vi "Lab Panel V6.00.vi"() -> ()   [LabVIEW 2017] (continued)
                            n1487 = local write "DISP LAB03-1"(w2783) -> ()
                          }
                        }
                      }
                      frame False {
                      }
                    }
                  }
                }
              }
              frame #5 {
                # "LAB03-2"
                n1488 = Equal?(x=w2786, y=2) -> (x = y?=w2789:bool)
                n1489 = local read "DISP LAB03-2"() -> (w2791:T4)
                n1490 = Unbundle(w2791) -> ("STATUS"=w2792:string)  [unwired: 2 out]
                n1491 = Equal?(x=w2792, y="RUN") -> (x = y?=w2788:bool)
                n1492 = And(x=w2788, y=w2789) -> (x .and. y?=w2787:bool)
                n1493 = case shown="True" w2787 {
                  tunnel: w2791 -> [_ w2795]
                  tunnel: w2785 -> [_ w2798]
                  frame False {
                  }
                  frame True {
                    n1494 = local read "SET LAB03-2"() -> (w2797:T5)
                    n1495 = local read "TDMS LAB03-2"() -> (w2794:refnum<k34>)
                    n1496 = Unbundle(w2795) -> ("CYCLE"=w2799:dbl)  [unwired: 2 out]
                    n1497 = Unbundle(w2797) -> ("T-RISE mins"=w2796:dbl)  [unwired: 4 out]
                    n1498 = Greater Or Equal?(x=w2799, y=w2798) -> (x >= y?=w2800:bool)
                    n1499 = case shown="True" w2800 {
                      tunnel: w2796 -> [w2803 _]
                      tunnel: w2795 -> [w2802 _]
                      tunnel: w2794 -> [w2801 _]
                      frame True {
                        n1500 = stacked-sequence {
                          tunnel: w2803 -> [w2806 _]
                          tunnel: w2802 -> [_ w2811]
                          tunnel: w2801 -> [w2804 _]
                          frame #0 {
                            n1501 = Build Array("T-RISE") -> (w2808:string[])
                            n1502 = Build Array(w2806) -> (w2807:dbl[])
                            n1503 = TDMS Write(0:w2804, 5:"TEST PASS", 7:w2808, 9:w2807) -> (15:w2810:errorcluster)  [unwired: 2 in, 3 out]
                            n1504 = local write "data file error"(w2810) -> ()
                          }
                          frame #1 {
                            n1505 = Bundle(cluster=w2811, "STATUS"="T-RISE PASS") -> (w2813:T4)  [unwired: 2 in]
                            n1506 = local write "RESULT LAB03-2"(TRUE) -> ()
                            n1507 = local write "DISP LAB03-2"(w2813) -> ()
                          }
                        }
                      }
                      frame False {
                      }
                    }
                  }
                }
              }
              frame #6 {
                # "LAB04-1"
                n1508 = Equal?(x=w2816, y=2) -> (x = y?=w2819:bool)
                n1509 = local read "DISP LAB04-1"() -> (w2821:T4)
                n1510 = Unbundle(w2821) -> ("STATUS"=w2822:string)  [unwired: 2 out]
                n1511 = Equal?(x=w2822, y="RUN") -> (x = y?=w2818:bool)
                n1512 = And(x=w2818, y=w2819) -> (x .and. y?=w2817:bool)
                n1513 = case shown="True" w2817 {
                  tunnel: w2821 -> [_ w2825]
                  tunnel: w2815 -> [_ w2828]
                  frame False {
                  }
                  frame True {
                    n1514 = local read "SET LAB04-1"() -> (w2827:T5)
                    n1515 = local read "TDMS LAB04-1"() -> (w2824:refnum<k34>)
                    n1516 = Unbundle(w2825) -> ("CYCLE"=w2829:dbl)  [unwired: 2 out]
                    n1517 = Unbundle(w2827) -> ("T-RISE mins"=w2826:dbl)  [unwired: 4 out]
                    n1518 = Greater Or Equal?(x=w2829, y=w2828) -> (x >= y?=w2830:bool)
                    n1519 = case shown="True" w2830 {
                      tunnel: w2826 -> [w2833 _]
                      tunnel: w2825 -> [w2832 _]
                      tunnel: w2824 -> [w2831 _]
                      frame True {
                        n1520 = stacked-sequence {
                          tunnel: w2833 -> [w2836 _]
                          tunnel: w2832 -> [_ w2841]
                          tunnel: w2831 -> [w2834 _]
                          frame #0 {
                            n1521 = Build Array("T-RISE") -> (w2838:string[])
                            n1522 = Build Array(w2836) -> (w2837:dbl[])
                            n1523 = TDMS Write(0:w2834, 5:"TEST PASS", 7:w2838, 9:w2837) -> (15:w2840:errorcluster)  [unwired: 2 in, 3 out]
                            n1524 = local write "data file error"(w2840) -> ()
                          }
                          frame #1 {
                            n1525 = Bundle(cluster=w2841, "STATUS"="T-RISE PASS") -> (w2843:T4)  [unwired: 2 in]
                            n1526 = local write "RESULT LAB04-1"(TRUE) -> ()
                            n1527 = local write "DISP LAB04-1"(w2843) -> ()
                          }
                        }
                      }
                      frame False {
                      }
                    }
                  }
                }
              }
              frame #7 {
                # "LAB04-2"
                n1528 = Equal?(x=w2846, y=2) -> (x = y?=w2849:bool)
                n1529 = local read "DISP LAB04-2"() -> (w2851:T4)
                n1530 = Unbundle(w2851) -> ("STATUS"=w2852:string)  [unwired: 2 out]
                n1531 = Equal?(x=w2852, y="RUN") -> (x = y?=w2848:bool)
                n1532 = And(x=w2848, y=w2849) -> (x .and. y?=w2847:bool)
                n1533 = case shown="True" w2847 {
                  tunnel: w2851 -> [_ w2855]
                  tunnel: w2845 -> [_ w2858]
                  frame False {
                  }
                  frame True {
                    n1534 = local read "SET LAB04-2"() -> (w2857:T5)
                    n1535 = local read "TDMS LAB04-2"() -> (w2854:refnum<k34>)
                    n1536 = Unbundle(w2855) -> ("CYCLE"=w2859:dbl)  [unwired: 2 out]
                    n1537 = Unbundle(w2857) -> ("T-RISE mins"=w2856:dbl)  [unwired: 4 out]
                    n1538 = Greater Or Equal?(x=w2859, y=w2858) -> (x >= y?=w2860:bool)
                    n1539 = case shown="True" w2860 {
                      tunnel: w2856 -> [w2863 _]
                      tunnel: w2855 -> [w2862 _]
                      tunnel: w2854 -> [w2861 _]
                      frame True {
                        n1540 = stacked-sequence {
                          tunnel: w2863 -> [w2866 _]
                          tunnel: w2862 -> [_ w2871]
                          tunnel: w2861 -> [w2864 _]
                          frame #0 {
                            n1541 = Build Array("T-RISE") -> (w2868:string[])
                            n1542 = Build Array(w2866) -> (w2867:dbl[])
                            n1543 = TDMS Write(0:w2864, 5:"TEST PASS", 7:w2868, 9:w2867) -> (15:w2870:errorcluster)  [unwired: 2 in, 3 out]
                            n1544 = local write "data file error"(w2870) -> ()
                          }
                          frame #1 {
                            n1545 = Bundle(cluster=w2871, "STATUS"="T-RISE PASS") -> (w2873:T4)  [unwired: 2 in]
                            n1546 = local write "RESULT LAB04-2"(TRUE) -> ()
                            n1547 = local write "DISP LAB04-2"(w2873) -> ()
                          }
                        }
                      }
                      frame False {
                      }
                    }
                  }
                }
              }
              frame #8 {
                # "LAB05-1"
                n1548 = Equal?(x=w2876, y=2) -> (x = y?=w2879:bool)
                n1549 = local read "DISP LAB05-1"() -> (w2881:T4)
                n1550 = Unbundle(w2881) -> ("STATUS"=w2882:string)  [unwired: 2 out]
                n1551 = Equal?(x=w2882, y="RUN") -> (x = y?=w2878:bool)
                n1552 = And(x=w2878, y=w2879) -> (x .and. y?=w2877:bool)
                n1553 = case shown="True" w2877 {
                  tunnel: w2881 -> [_ w2885]
                  tunnel: w2875 -> [_ w2888]
                  frame False {
                  }
                  frame True {
                    n1554 = local read "SET LAB05-1"() -> (w2887:T5)
                    n1555 = local read "TDMS LAB05-1"() -> (w2884:refnum<k34>)
                    n1556 = Unbundle(w2885) -> ("CYCLE"=w2889:dbl)  [unwired: 2 out]
                    n1557 = Unbundle(w2887) -> ("T-RISE mins"=w2886:dbl)  [unwired: 4 out]
                    n1558 = Greater Or Equal?(x=w2889, y=w2888) -> (x >= y?=w2890:bool)
                    n1559 = case shown="True" w2890 {
                      tunnel: w2886 -> [w2893 _]
                      tunnel: w2885 -> [w2892 _]
                      tunnel: w2884 -> [w2891 _]
                      frame True {
                        n1560 = stacked-sequence {
                          tunnel: w2893 -> [w2896 _]
                          tunnel: w2892 -> [_ w2901]
                          tunnel: w2891 -> [w2894 _]
                          frame #0 {
                            n1561 = Build Array("T-RISE") -> (w2898:string[])
                            n1562 = Build Array(w2896) -> (w2897:dbl[])
                            n1563 = TDMS Write(0:w2894, 5:"TEST PASS", 7:w2898, 9:w2897) -> (15:w2900:errorcluster)  [unwired: 2 in, 3 out]
                            n1564 = local write "data file error"(w2900) -> ()
                          }
                          frame #1 {
                            n1565 = Bundle(cluster=w2901, "STATUS"="T-RISE PASS") -> (w2903:T4)  [unwired: 2 in]
                            n1566 = local write "RESULT LAB05-1"(TRUE) -> ()
                            n1567 = local write "DISP LAB05-1"(w2903) -> ()
                          }
                        }
                      }
                      frame False {
                      }
                    }
                  }
                }
              }
              frame #9 {
                # "LAB05-2"
                n1568 = Equal?(x=w2906, y=2) -> (x = y?=w2909:bool)
                n1569 = local read "DISP LAB05-2"() -> (w2911:T4)
                n1570 = Unbundle(w2911) -> ("STATUS"=w2912:string)  [unwired: 2 out]
                n1571 = Equal?(x=w2912, y="RUN") -> (x = y?=w2908:bool)
                n1572 = And(x=w2908, y=w2909) -> (x .and. y?=w2907:bool)
                n1573 = case shown="True" w2907 {
                  tunnel: w2911 -> [_ w2915]
                  tunnel: w2905 -> [_ w2918]
                  frame False {
                  }
                  frame True {
                    n1574 = local read "SET LAB05-2"() -> (w2917:T5)
                    n1575 = local read "TDMS LAB05-2"() -> (w2914:refnum<k34>)
                    n1576 = Unbundle(w2915) -> ("CYCLE"=w2919:dbl)  [unwired: 2 out]
                    n1577 = Unbundle(w2917) -> ("T-RISE mins"=w2916:dbl)  [unwired: 4 out]
                    n1578 = Greater Or Equal?(x=w2919, y=w2918) -> (x >= y?=w2920:bool)
                    n1579 = case shown="True" w2920 {
                      tunnel: w2916 -> [w2923 _]
                      tunnel: w2915 -> [w2922 _]
                      tunnel: w2914 -> [w2921 _]
                      frame True {
                        n1580 = stacked-sequence {
                          tunnel: w2923 -> [w2926 _]
                          tunnel: w2922 -> [_ w2931]
                          tunnel: w2921 -> [w2924 _]
                          frame #0 {
                            n1581 = Build Array("T-RISE") -> (w2928:string[])
                            n1582 = Build Array(w2926) -> (w2927:dbl[])
                            n1583 = TDMS Write(0:w2924, 5:"TEST PASS", 7:w2928, 9:w2927) -> (15:w2930:errorcluster)  [unwired: 2 in, 3 out]
                            n1584 = local write "data file error"(w2930) -> ()
                          }
                          frame #1 {
                            n1585 = Bundle(cluster=w2931, "STATUS"="T-RISE PASS") -> (w2933:T4)  [unwired: 2 in]
                            n1586 = local write "RESULT LAB05-2"(TRUE) -> ()
                            n1587 = local write "DISP LAB05-2"(w2933) -> ()
                          }
                        }
                      }
                      frame False {
                      }
                    }
                  }
                }
              }
            }
          }
          frame #7 {
            # "Note : run lab0X-N. RUN LAB0X-N and O/I LAB0X-N   are written to digital I/O in frame 11"
            # "End test & close test files"
            n1588 = local read "MAIL SETTINGS"() -> (w2940:T7)
            n1589 = local read "TO (string):"() -> (w2935:string)
            n1590 = Unbundle(w2940) -> ("OUT SERVER ADDRESS"=w2939:string, "FROM ACCOUNT"=w2938:string)  [unwired: 5 out]
            n1591 = stacked-sequence {
              tunnel: w2950 -> [_ _ _ _ _ _ _ _ _ _]
              tunnel: w2951 -> [_ _ _ _ _ _ _ _ _ _]
              tunnel: w2949 -> [_ _ _ _ _ _ _ _ _ _]
              tunnel: w2948 -> [_ _ _ _ _ _ _ _ _ _]
              tunnel: w2947 -> [_ _ _ _ _ _ _ _ _ _]
              tunnel: w2946 -> [_ _ _ _ _ _ _ _ _ _]
              tunnel: w2945 -> [_ _ _ _ _ _ _ _ _ _]
              tunnel: w2944 -> [_ _ _ _ _ _ _ _ _ _]
              tunnel: w2943 -> [_ _ _ _ _ _ _ _ _ _]
              tunnel: w2942 -> [_ _ _ _ _ _ _ _ _ _]
              tunnel: w2939 -> [w2956 w3008 w3056 w3103 w3150 w3197 w3244 w3291 w3338 w3385]
              tunnel: w2938 -> [w2955 w3007 w3055 w3102 w3149 w3196 w3243 w3290 w3337 w3384]
              tunnel: "Mail Test File To:" -> [w2954 w3006 w3054 w3101 w3148 w3195 w3242 w3289 w3336 w3383]
              tunnel: "Mail Test Fail" -> [w2953 w3005 w3053 w3100 w3147 w3194 w3241 w3288 w3335 w3382]
              frame #0 {
                # "LAB01-1"
                n1592 = local read "DISP LAB01-1"() -> (w2952:T4)
                n1593 = global write "Global display 2.vi" "DISP LAB01-1"(w2952) -> ()
                n1594 = local read "run lab01-1"() -> (w2957:bool)
                n1595 = local read "TDMS LAB01-1"() -> (w2958:refnum<k34>)
                n1596 = Unbundle(w2952) -> ("CYCLE"=w2960:dbl, "STATUS"=w2959:string)  [unwired: 1 out]
                n1597 = case shown="True" w2957 {
                  tunnel: w2960 -> [_ w2966]
                  tunnel: w2952 -> [_ w2968]
                  tunnel: w2959 -> [_ w2965]
                  tunnel: w2958 -> [_ w2967]
                  tunnel: w2956 -> [_ w2964]
                  tunnel: w2955 -> [_ w2963]
                  tunnel: w2954 -> [_ w2962]
                  tunnel: w2953 -> [_ w2961]
                  frame False {
                  }
                  frame True {
                    n1598 = Not Equal?(x=w2965, y="RUN") -> (x != y?=w2969:bool)
                    n1599 = Greater?(x=w2966, y=2.0) -> (0:w2971:bool)
                    n1600 = And(x=w2971, y=w2969) -> (x .and. y?=w2970:bool)
                    n1601 = case shown="True" w2970 {
                      tunnel: w2968 -> [_ w2981]
                      tunnel: w2967 -> [_ w2980]
                      tunnel: w2966 -> [_ w2979]
                      tunnel: w2965 -> [_ w2978]
                      tunnel: w2964 -> [_ w2977]
                      tunnel: w2963 -> [_ w2976]
                      tunnel: w2962 -> [_ w2975]
                      tunnel: w2961 -> [_ w2974]
                      frame False {
                      }
                      frame True {
                        n1602 = stacked-sequence {
                          tunnel: w2981 -> [w2985 _ _]
                          tunnel: w2980 -> [_ w2987 _]
                          tunnel: w2979 -> [_ _ _]
                          tunnel: w2978 -> [_ _ w2993]
                          tunnel: w2977 -> [_ _ w2992]
                          tunnel: w2976 -> [_ _ w2991]
                          tunnel: w2975 -> [_ _ w2990]
                          tunnel: w2974 -> [_ _ w2989]
                          frame #0 {
                            w2982 = FALSE
                            n1603 = local write "mail control"("END") -> ()
                            n1604 = Bundle(cluster=w2985) -> (w2984:T4)  [unwired: 3 in]
                            n1605 = local write "DISP LAB01-1"(w2984) -> ()
                            n1606 = local write "O/I  LAB01-1"(w2982) -> ()
                            n1607 = local write "run lab01-1"(w2982) -> ()
                            n1608 = local write "RUN LAB01-1"(w2982) -> ()
                          }
                          frame #1 {
                            n1609 = TDMS Close(11:w2987) -> (0:w2986:errorcluster)  [unwired: 1 in, 1 out]
                            n1610 = local write "data file error"(w2986) -> ()
                          }
                          frame #2 {
                            n1611 = stacked-sequence {
                              tunnel: "LAB01-1" -> [w2995 w2998 _]
                              tunnel: w2993 -> [_ w3004 _]
                              tunnel: w2992 -> [_ w3003 _]
                              tunnel: w2991 -> [_ w3002 _]
                              tunnel: w2990 -> [_ w3001 _]
                              tunnel: w2989 -> [_ w3000 _]
                              frame #0 {
                                n1612 = call "sub vi - defrag tdms v1.vi"("panel id"=w2995) -> ("error out"=w2994:errorcluster)  [unwired: 10 in]
                                n1613 = local write "data file error"(w2994) -> ()
                              }
                              frame #1 {
                                n1614 = Bundle By Name(cluster=T24 {"status"="", "mail server"="", "mail from"="", "mail to"="", "mail file"=FALSE} ("Input Cluster"), "status"=w3004, "mail server"=w3003, "mail from"=w3002, "mail to"=w3001, "mail file"=w3000) -> (w2997:T24)
                                n1615 = call "Save data file (pass-fail) v5.vi"("Input Cluster"=w2997, "panel id"=w2998) -> ("network file save error"=w2999:errorcluster)  [unwired: 8 in, 1 out]
                                n1616 = local write "data file error"(w2999) -> ()
                              }
                              frame #2 {
                              }
                            }
                          }
                        }
                      }
                    }
                  }
                }
              }
              frame #1 {
                # "LAB01-2"
                n1617 = local read "run lab01-2"() -> (w3009:bool)
                n1618 = case shown="True" w3009 {
                  tunnel: w3008 -> [_ w3014]
                  tunnel: w3007 -> [_ w3013]
                  tunnel: w3006 -> [_ w3012]
                  tunnel: w3005 -> [_ w3011]
                  frame False {
                  }
                  frame True {
                    n1619 = local read "DISP LAB01-2"() -> (w3010:T4)
                    n1620 = global write "Global display 2.vi" "DISP LAB01-2"(w3010) -> ()
                    n1621 = local read "TDMS LAB01-2"() -> (w3021:refnum<k34>)
                    n1622 = Unbundle(w3010) -> ("CYCLE"=w3016:dbl, "STATUS"=w3015:string)  [unwired: 1 out]
                    n1623 = Not Equal?(x=w3015, y="RUN") -> (x != y?=w3018:bool)
                    n1624 = Greater?(x=w3016, y=2.0) -> (0:w3019:bool)
                    n1625 = And(x=w3019, y=w3018) -> (x .and. y?=w3017:bool)
                    n1626 = case shown="True" w3017 {
                      tunnel: w3010 -> [_ w3030]
                      tunnel: w3021 -> [_ w3029]
                      tunnel: w3016 -> [_ w3028]
                      tunnel: w3015 -> [_ w3027]
                      tunnel: w3014 -> [_ w3026]
                      tunnel: w3013 -> [_ w3025]
                      tunnel: w3012 -> [_ w3024]
                      tunnel: w3011 -> [_ w3023]
                      frame False {
                      }
                      frame True {
                        n1627 = stacked-sequence {
                          tunnel: w3030 -> [w3033 _ _]
                          tunnel: w3029 -> [_ w3035 _]
                          tunnel: w3028 -> [_ _ _]
                          tunnel: w3027 -> [_ _ w3041]
                          tunnel: w3026 -> [_ _ w3040]
                          tunnel: w3025 -> [_ _ w3039]
                          tunnel: w3024 -> [_ _ w3038]
                          tunnel: w3023 -> [_ _ w3037]
                          frame #0 {
                            w3031 = FALSE
                            n1628 = local write "mail control"("END") -> ()
                            n1629 = Bundle(cluster=w3033) -> (w3034:T4)  [unwired: 3 in]
                            n1630 = local write "RUN LAB01-2"(w3031) -> ()
                            n1631 = local write "run lab01-2"(w3031) -> ()
                            n1632 = local write "O/I  LAB01-2"(w3031) -> ()
                            n1633 = local write "DISP LAB01-2"(w3034) -> ()
                          }
                          frame #1 {
                            n1634 = TDMS Close(11:w3035) -> (0:w3036:errorcluster)  [unwired: 1 in, 1 out]
                            n1635 = local write "data file error"(w3036) -> ()
                          }
                          frame #2 {
                            n1636 = stacked-sequence {
                              tunnel: "LAB01-2" -> [w3044 w3045]
                              tunnel: w3041 -> [_ w3050]
                              tunnel: w3040 -> [_ w3049]
                              tunnel: w3039 -> [_ w3048]
                              tunnel: w3038 -> [_ w3047]
                              tunnel: w3037 -> [_ w3046]
                              frame #0 {
                                n1637 = call "sub vi - defrag tdms v1.vi"("panel id"=w3044) -> ("error out"=w3043:errorcluster)  [unwired: 10 in]
                                n1638 = local write "data file error"(w3043) -> ()
                              }
                              frame #1 {
                                n1639 = Bundle("STATUS"=w3050, "OUT SERVER ADDRESS"=w3049, "FROM ACCOUNT"=w3048, "Mail Test File To:"=w3047, "Mail Test Fail"=w3046) -> (w3052:T32)  [unwired: 1 in]
                                n1640 = call "Save data file (pass-fail) v5.vi"("Input Cluster"=w3052, "panel id"=w3045) -> ("network file save error"=w3051:errorcluster)  [unwired: 8 in, 1 out]
                                n1641 = local write "data file error"(w3051) -> ()
                              }
                            }
                          }
                        }
                      }
                    }
                  }
                }
              }
              frame #2 {
                # "LAB02-1"
                n1642 = local read "run lab02-1"() -> (w3057:bool)
                n1643 = case shown="True" w3057 {
                  tunnel: w3056 -> [_ w3062]
                  tunnel: w3055 -> [_ w3061]
                  tunnel: w3054 -> [_ w3060]
                  tunnel: w3053 -> [_ w3059]
                  frame False {
                  }
                  frame True {
                    n1644 = local read "DISP LAB02-1"() -> (w3058:T4)
                    n1645 = global write "Global display 2.vi" "DISP LAB02-1"(w3058) -> ()
                    n1646 = Unbundle(w3058) -> ("CYCLE"=w3066:dbl, "STATUS"=w3063:string)  [unwired: 1 out]
                    n1647 = local read "TDMS LAB02-1"() -> (w3069:refnum<k34>)
                    n1648 = Not Equal?(x=w3063, y="RUN") -> (x != y?=w3065:bool)
                    n1649 = Greater?(x=w3066, y=2.0) -> (0:w3067:bool)
                    n1650 = And(x=w3067, y=w3065) -> (x .and. y?=w3064:bool)
                    n1651 = case shown="True" w3064 {
                      tunnel: w3058 -> [_ w3077]
                      tunnel: w3069 -> [_ w3076]
                      tunnel: w3063 -> [_ w3075]
                      tunnel: w3062 -> [_ w3074]
                      tunnel: w3061 -> [_ w3073]
                      tunnel: w3060 -> [_ w3072]
                      tunnel: w3059 -> [_ w3071]
                      frame False {
                      }
                      frame True {
                        n1652 = stacked-sequence {
                          tunnel: w3077 -> [w3080 _ _]
                          tunnel: w3076 -> [_ w3082 _]
                          tunnel: w3075 -> [_ _ w3088]
                          tunnel: w3074 -> [_ _ w3087]
                          tunnel: w3073 -> [_ _ w3086]
                          tunnel: w3072 -> [_ _ w3085]
                          tunnel: w3071 -> [_ _ w3084]
                          frame #0 {
                            w3078 = FALSE
                            n1653 = local write "mail control"("END") -> ()
                            n1654 = Bundle(cluster=w3080) -> (w3081:T4)  [unwired: 3 in]
                            n1655 = local write "O/I  LAB02-1"(w3078) -> ()
                            n1656 = local write "RUN LAB02-1"(w3078) -> ()
                            n1657 = local write "run lab02-1"(w3078) -> ()
                            n1658 = local write "DISP LAB02-1"(w3081) -> ()
                          }
                          frame #1 {
                            n1659 = TDMS Close(11:w3082) -> (0:w3083:errorcluster)  [unwired: 1 in, 1 out]
                            n1660 = local write "data file error"(w3083) -> ()
                          }
                          frame #2 {
                            n1661 = stacked-sequence {
                              tunnel: "LAB02-1" -> [w3091 w3098]
                              tunnel: w3088 -> [_ w3096]
                              tunnel: w3087 -> [_ w3095]
                              tunnel: w3086 -> [_ w3094]
                              tunnel: w3085 -> [_ w3093]
                              tunnel: w3084 -> [_ w3092]
                              frame #0 {
                                n1662 = call "sub vi - defrag tdms v1.vi"("panel id"=w3091) -> ("error out"=w3090:errorcluster)  [unwired: 10 in]
                                n1663 = local write "data file error"(w3090) -> ()
                              }
                              frame #1 {
                                n1664 = Bundle("STATUS"=w3096, "OUT SERVER ADDRESS"=w3095, "FROM ACCOUNT"=w3094, "Mail Test File To:"=w3093, "Mail Test Fail"=w3092) -> (w3097:T32)  [unwired: 1 in]
                                n1665 = call "Save data file (pass-fail) v5.vi"("Input Cluster"=w3097, "panel id"=w3098) -> ("network file save error"=w3099:errorcluster)  [unwired: 8 in, 1 out]
                                n1666 = local write "data file error"(w3099) -> ()
                              }
                            }
                          }
                        }
                      }
                    }
                  }
                }
              }
              frame #3 {
                # "LAB02-2"
                n1667 = local read "run lab02-2"() -> (w3104:bool)
                n1668 = case shown="True" w3104 {
                  tunnel: w3103 -> [_ w3110]
                  tunnel: w3102 -> [_ w3109]
                  tunnel: w3101 -> [_ w3108]
                  tunnel: w3100 -> [_ w3107]
                  frame False {
                  }
                  frame True {
                    n1669 = local read "DISP LAB02-2"() -> (w3106:T4)
                    n1670 = global write "Global display 2.vi" "DISP LAB02-2"(w3106) -> ()
                    n1671 = local read "TDMS LAB02-2"() -> (w3116:refnum<k34>)
                    n1672 = Unbundle(w3106) -> ("CYCLE"=w3105:dbl, "STATUS"=w3111:string)  [unwired: 1 out]
                    n1673 = Not Equal?(x=w3111, y="RUN") -> (x != y?=w3113:bool)
                    n1674 = Greater?(x=w3105, y=2.0) -> (0:w3114:bool)
                    n1675 = And(x=w3114, y=w3113) -> (x .and. y?=w3112:bool)
                    n1676 = case shown="True" w3112 {
                      tunnel: w3106 -> [_ w3124]
                      tunnel: w3116 -> [_ w3123]
                      tunnel: w3111 -> [_ w3122]
                      tunnel: w3110 -> [_ w3121]
                      tunnel: w3109 -> [_ w3120]
                      tunnel: w3108 -> [_ w3119]
                      tunnel: w3107 -> [_ w3118]
                      frame False {
                      }
                      frame True {
                        n1677 = stacked-sequence {
                          tunnel: w3124 -> [w3127 _ _]
                          tunnel: w3123 -> [_ w3129 _]
                          tunnel: w3122 -> [_ _ w3135]
                          tunnel: w3121 -> [_ _ w3134]
                          tunnel: w3120 -> [_ _ w3133]
                          tunnel: w3119 -> [_ _ w3132]
                          tunnel: w3118 -> [_ _ w3131]
                          frame #0 {
                            w3125 = FALSE
                            n1678 = local write "mail control"("END") -> ()
                            n1679 = Bundle(cluster=w3127) -> (w3128:T4)  [unwired: 3 in]
                            n1680 = local write "O/I  LAB02-2"(w3125) -> ()
                            n1681 = local write "run lab02-2"(w3125) -> ()
                            n1682 = local write "RUN LAB02-2"(w3125) -> ()
                            n1683 = local write "DISP LAB02-2"(w3128) -> ()
                          }
                          frame #1 {
                            n1684 = TDMS Close(11:w3129) -> (0:w3130:errorcluster)  [unwired: 1 in, 1 out]
                            n1685 = local write "data file error"(w3130) -> ()
                          }
                          frame #2 {
                            n1686 = stacked-sequence {
                              tunnel: "LAB02-2" -> [w3138 w3144]
                              tunnel: w3135 -> [_ w3143]
                              tunnel: w3134 -> [_ w3142]
                              tunnel: w3133 -> [_ w3141]
                              tunnel: w3132 -> [_ w3140]
                              tunnel: w3131 -> [_ w3139]
                              frame #0 {
                                n1687 = call "sub vi - defrag tdms v1.vi"("panel id"=w3138) -> ("error out"=w3137:errorcluster)  [unwired: 10 in]
                                n1688 = local write "data file error"(w3137) -> ()
                              }
                              frame #1 {
                                n1689 = Bundle("STATUS"=w3143, "OUT SERVER ADDRESS"=w3142, "FROM ACCOUNT"=w3141, "Mail Test File To:"=w3140, "Mail Test Fail"=w3139) -> (w3146:T32)  [unwired: 1 in]
                                n1690 = call "Save data file (pass-fail) v5.vi"("Input Cluster"=w3146, "panel id"=w3144) -> ("network file save error"=w3145:errorcluster)  [unwired: 8 in, 1 out]
                                n1691 = local write "data file error"(w3145) -> ()
                              }
                            }
                          }
                        }
                      }
                    }
                  }
                }
              }
              frame #4 {
                # "LAB03-1"
                n1692 = local read "run lab03-1"() -> (w3151:bool)
                n1693 = case shown="True" w3151 {
                  tunnel: w3150 -> [_ w3156]
                  tunnel: w3149 -> [_ w3155]
                  tunnel: w3148 -> [_ w3154]
                  tunnel: w3147 -> [_ w3153]
                  frame False {
                  }
                  frame True {
                    n1694 = local read "DISP LAB03-1"() -> (w3152:T4)
                    n1695 = local read "TDMS LAB03-1"() -> (w3163:refnum<k34>)
                    n1696 = global write "Global display 2.vi" "DISP LAB03-1"(w3152) -> ()
                    n1697 = Unbundle(w3152) -> ("CYCLE"=w3160:dbl, "STATUS"=w3157:string)  [unwired: 1 out]
                    n1698 = Not Equal?(x=w3157, y="RUN") -> (x != y?=w3159:bool)
                    n1699 = Greater?(x=w3160, y=2.0) -> (0:w3161:bool)
                    n1700 = And(x=w3161, y=w3159) -> (x .and. y?=w3158:bool)
                    n1701 = case shown="True" w3158 {
                      tunnel: w3152 -> [_ w3171]
                      tunnel: w3163 -> [_ w3170]
                      tunnel: w3157 -> [_ w3169]
                      tunnel: w3156 -> [_ w3168]
                      tunnel: w3155 -> [_ w3167]
                      tunnel: w3154 -> [_ w3166]
                      tunnel: w3153 -> [_ w3165]
                      frame False {
                      }
                      frame True {
                        n1702 = stacked-sequence {
                          tunnel: w3171 -> [w3174 _ _]
                          tunnel: w3170 -> [_ w3176 _]
                          tunnel: w3169 -> [_ _ w3182]
                          tunnel: w3168 -> [_ _ w3181]
                          tunnel: w3167 -> [_ _ w3180]
                          tunnel: w3166 -> [_ _ w3179]
                          tunnel: w3165 -> [_ _ w3178]
                          frame #0 {
                            w3172 = FALSE
                            n1703 = local write "mail control"("END") -> ()
                            n1704 = Bundle(cluster=w3174) -> (w3175:T4)  [unwired: 3 in]
                            n1705 = local write "O/I  LAB03-1"(w3172) -> ()
                            n1706 = local write "run lab03-1"(w3172) -> ()
                            n1707 = local write "RUN LAB03-1"(w3172) -> ()
                            n1708 = local write "DISP LAB03-1"(w3175) -> ()
                          }
                          frame #1 {
                            n1709 = TDMS Close(11:w3176) -> (0:w3177:errorcluster)  [unwired: 1 in, 1 out]
                            n1710 = local write "data file error"(w3177) -> ()
                          }
                          frame #2 {
                            n1711 = stacked-sequence {
                              tunnel: "LAB03-1" -> [w3185 w3191]
                              tunnel: w3182 -> [_ w3190]
                              tunnel: w3181 -> [_ w3189]
                              tunnel: w3180 -> [_ w3188]
                              tunnel: w3179 -> [_ w3187]
                              tunnel: w3178 -> [_ w3186]
                              frame #0 {
                                n1712 = call "sub vi - defrag tdms v1.vi"("panel id"=w3185) -> ("error out"=w3184:errorcluster)  [unwired: 10 in]
                                n1713 = local write "data file error"(w3184) -> ()
                              }
                              frame #1 {
                                n1714 = Bundle("STATUS"=w3190, "OUT SERVER ADDRESS"=w3189, "FROM ACCOUNT"=w3188, "Mail Test File To:"=w3187, "Mail Test Fail"=w3186) -> (w3193:T32)  [unwired: 1 in]
                                n1715 = call "Save data file (pass-fail) v5.vi"("Input Cluster"=w3193, "panel id"=w3191) -> ("network file save error"=w3192:errorcluster)  [unwired: 8 in, 1 out]
                                n1716 = local write "data file error"(w3192) -> ()
                              }
                            }
                          }
                        }
                      }
                    }
                  }
                }
              }
              frame #5 {
                # "LAB03-2"
                n1717 = local read "run lab03-2"() -> (w3198:bool)
                n1718 = case shown="True" w3198 {
                  tunnel: w3197 -> [_ w3203]
                  tunnel: w3196 -> [_ w3202]
                  tunnel: w3195 -> [_ w3201]
                  tunnel: w3194 -> [_ w3200]
                  frame False {
                  }
                  frame True {
                    n1719 = local read "DISP LAB03-2"() -> (w3199:T4)
                    n1720 = global write "Global display 2.vi" "DISP LAB03-2"(w3199) -> ()
                    n1721 = Unbundle(w3199) -> ("CYCLE"=w3207:dbl, "STATUS"=w3204:string)  [unwired: 1 out]
                    n1722 = local read "TDMS LAB03-2"() -> (w3210:refnum<k34>)
                    n1723 = Not Equal?(x=w3204, y="RUN") -> (x != y?=w3206:bool)
                    n1724 = Greater?(x=w3207, y=2.0) -> (0:w3208:bool)
                    n1725 = And(x=w3208, y=w3206) -> (x .and. y?=w3205:bool)
                    n1726 = case shown="True" w3205 {
                      tunnel: w3199 -> [_ w3218]
                      tunnel: w3210 -> [_ w3217]
                      tunnel: w3204 -> [_ w3216]
                      tunnel: w3203 -> [_ w3215]
                      tunnel: w3202 -> [_ w3214]
                      tunnel: w3201 -> [_ w3213]
                      tunnel: w3200 -> [_ w3212]
                      frame False {
                      }
                      frame True {
                        n1727 = stacked-sequence {
                          tunnel: w3218 -> [w3221 _ _]
                          tunnel: w3217 -> [_ w3223 _]
                          tunnel: w3216 -> [_ _ w3229]
                          tunnel: w3215 -> [_ _ w3228]
                          tunnel: w3214 -> [_ _ w3227]
                          tunnel: w3213 -> [_ _ w3226]
                          tunnel: w3212 -> [_ _ w3225]
                          frame #0 {
                            w3219 = FALSE
                            n1728 = local write "mail control"("END") -> ()
                            n1729 = Bundle(cluster=w3221) -> (w3222:T4)  [unwired: 3 in]
                            n1730 = local write "RUN LAB03-2"(w3219) -> ()
                            n1731 = local write "O/I  LAB03-2"(w3219) -> ()
                            n1732 = local write "DISP LAB03-2"(w3222) -> ()
                            n1733 = local write "run lab03-2"(w3219) -> ()
                          }
                          frame #1 {
                            n1734 = TDMS Close(11:w3223) -> (0:w3224:errorcluster)  [unwired: 1 in, 1 out]
                            n1735 = local write "data file error"(w3224) -> ()
                          }
                          frame #2 {
                            n1736 = stacked-sequence {
                              tunnel: "LAB03-2" -> [w3232 w3233]
                              tunnel: w3229 -> [_ w3238]
                              tunnel: w3228 -> [_ w3237]
                              tunnel: w3227 -> [_ w3236]
                              tunnel: w3226 -> [_ w3235]
                              tunnel: w3225 -> [_ w3234]
                              frame #0 {
                                n1737 = call "sub vi - defrag tdms v1.vi"("panel id"=w3232) -> ("error out"=w3231:errorcluster)  [unwired: 10 in]
                                n1738 = local write "data file error"(w3231) -> ()
                              }
                              frame #1 {
                                n1739 = Bundle("STATUS"=w3238, "OUT SERVER ADDRESS"=w3237, "FROM ACCOUNT"=w3236, "Mail Test File To:"=w3235, "Mail Test Fail"=w3234) -> (w3240:T32)  [unwired: 1 in]
                                n1740 = call "Save data file (pass-fail) v5.vi"("Input Cluster"=w3240, "panel id"=w3233) -> ("network file save error"=w3239:errorcluster)  [unwired: 8 in, 1 out]
                                n1741 = local write "data file error"(w3239) -> ()
                              }
                            }
                          }
                        }
                      }
                    }
                  }
                }
              }
              frame #6 {
                # "LAB04-1"
                n1742 = local read "run lab04-1"() -> (w3245:bool)
                n1743 = case shown="True" w3245 {
                  tunnel: w3244 -> [_ w3250]
                  tunnel: w3243 -> [_ w3249]
                  tunnel: w3242 -> [_ w3248]
                  tunnel: w3241 -> [_ w3247]
                  frame False {
                  }
                  frame True {
                    n1744 = local read "DISP LAB04-1"() -> (w3246:T4)
                    n1745 = Unbundle(w3246) -> ("CYCLE"=w3254:dbl, "STATUS"=w3251:string)  [unwired: 1 out]
                    n1746 = local read "TDMS LAB04-1"() -> (w3257:refnum<k34>)
                    n1747 = global write "Global display 2.vi" "DISP LAB04-1"(w3246) -> ()
                    n1748 = Not Equal?(x=w3251, y="RUN") -> (x != y?=w3253:bool)
                    n1749 = Greater?(x=w3254, y=2.0) -> (0:w3255:bool)
                    n1750 = And(x=w3255, y=w3253) -> (x .and. y?=w3252:bool)
                    n1751 = case shown="True" w3252 {
                      tunnel: w3246 -> [_ w3265]
                      tunnel: w3257 -> [_ w3264]
                      tunnel: w3251 -> [_ w3263]
                      tunnel: w3250 -> [_ w3262]
                      tunnel: w3249 -> [_ w3261]
                      tunnel: w3248 -> [_ w3260]
                      tunnel: w3247 -> [_ w3259]
                      frame False {
                      }
                      frame True {
                        n1752 = stacked-sequence {
                          tunnel: w3265 -> [w3268 _ _]
                          tunnel: w3264 -> [_ w3270 _]
                          tunnel: w3263 -> [_ _ w3276]
                          tunnel: w3262 -> [_ _ w3275]
                          tunnel: w3261 -> [_ _ w3274]
                          tunnel: w3260 -> [_ _ w3273]
                          tunnel: w3259 -> [_ _ w3272]
                          frame #0 {
                            w3266 = FALSE
                            n1753 = local write "mail control"("END") -> ()
                            n1754 = Bundle(cluster=w3268) -> (w3269:T4)  [unwired: 3 in]
                            n1755 = local write "RUN LAB04-1"(w3266) -> ()
                            n1756 = local write "O/I  LAB04-1"(w3266) -> ()
                            n1757 = local write "run lab04-1"(w3266) -> ()
                            n1758 = local write "DISP LAB04-1"(w3269) -> ()
                          }
                          frame #1 {
                            n1759 = TDMS Close(11:w3270) -> (0:w3271:errorcluster)  [unwired: 1 in, 1 out]
                            n1760 = local write "data file error"(w3271) -> ()
                          }
                          frame #2 {
                            n1761 = stacked-sequence {
                              tunnel: "LAB04-1" -> [w3279 w3280]
                              tunnel: w3276 -> [_ w3285]
                              tunnel: w3275 -> [_ w3284]
                              tunnel: w3274 -> [_ w3283]
                              tunnel: w3273 -> [_ w3282]
                              tunnel: w3272 -> [_ w3281]
                              frame #0 {
                                n1762 = call "sub vi - defrag tdms v1.vi"("panel id"=w3279) -> ("error out"=w3278:errorcluster)  [unwired: 10 in]
                                n1763 = local write "data file error"(w3278) -> ()
                              }
                              frame #1 {
                                n1764 = Bundle("STATUS"=w3285, "OUT SERVER ADDRESS"=w3284, "FROM ACCOUNT"=w3283, "Mail Test File To:"=w3282, "Mail Test Fail"=w3281) -> (w3287:T32)  [unwired: 1 in]
                                n1765 = call "Save data file (pass-fail) v5.vi"("Input Cluster"=w3287, "panel id"=w3280) -> ("network file save error"=w3286:errorcluster)  [unwired: 8 in, 1 out]
                                n1766 = local write "data file error"(w3286) -> ()
                              }
                            }
                          }
                        }
                      }
                    }
                  }
                }
              }
              frame #7 {
                # "LAB04-2"
                n1767 = local read "run lab04-2"() -> (w3292:bool)
                n1768 = case shown="True" w3292 {
                  tunnel: w3291 -> [_ w3297]
                  tunnel: w3290 -> [_ w3296]
                  tunnel: w3289 -> [_ w3295]
                  tunnel: w3288 -> [_ w3294]
                  frame False {
                  }
                  frame True {
                    n1769 = local read "DISP LAB04-2"() -> (w3293:T4)
                    n1770 = Unbundle(w3293) -> ("CYCLE"=w3301:dbl, "STATUS"=w3298:string)  [unwired: 1 out]
                    n1771 = global write "Global display 2.vi" "DISP LAB04-2"(w3293) -> ()
                    n1772 = Not Equal?(x=w3298, y="RUN") -> (x != y?=w3300:bool)
                    n1773 = local read "TDMS LAB04-2"() -> (w3304:refnum<k34>)
                    n1774 = Greater?(x=w3301, y=2.0) -> (0:w3302:bool)
                    n1775 = And(x=w3302, y=w3300) -> (x .and. y?=w3299:bool)
                    n1776 = case shown="True" w3299 {
                      tunnel: w3293 -> [_ w3312]
                      tunnel: w3304 -> [_ w3311]
                      tunnel: w3298 -> [_ w3310]
                      tunnel: w3297 -> [_ w3309]
                      tunnel: w3296 -> [_ w3308]
                      tunnel: w3295 -> [_ w3307]
                      tunnel: w3294 -> [_ w3306]
                      frame False {
                      }
                      frame True {
                        n1777 = stacked-sequence {
                          tunnel: w3312 -> [w3315 _ _]
                          tunnel: w3311 -> [_ w3317 _]
                          tunnel: w3310 -> [_ _ w3323]
                          tunnel: w3309 -> [_ _ w3322]
                          tunnel: w3308 -> [_ _ w3321]
                          tunnel: w3307 -> [_ _ w3320]
                          tunnel: w3306 -> [_ _ w3319]
                          frame #0 {
                            w3313 = FALSE
                            n1778 = local write "mail control"("END") -> ()
                            n1779 = Bundle(cluster=w3315) -> (w3316:T4)  [unwired: 3 in]
                            n1780 = local write "O/I  LAB04-2"(w3313) -> ()
                            n1781 = local write "RUN LAB04-2"(w3313) -> ()
                            n1782 = local write "run lab04-2"(w3313) -> ()
                            n1783 = local write "DISP LAB04-2"(w3316) -> ()
                          }
                          frame #1 {
                            n1784 = TDMS Close(11:w3317) -> (0:w3318:errorcluster)  [unwired: 1 in, 1 out]
                            n1785 = local write "data file error"(w3318) -> ()
                          }
                          frame #2 {
                            n1786 = stacked-sequence {
                              tunnel: "LAB04-2" -> [w3326 w3327]
                              tunnel: w3323 -> [_ w3332]
                              tunnel: w3322 -> [_ w3331]
                              tunnel: w3321 -> [_ w3330]
                              tunnel: w3320 -> [_ w3329]
                              tunnel: w3319 -> [_ w3328]
                              frame #0 {
                                n1787 = call "sub vi - defrag tdms v1.vi"("panel id"=w3326) -> ("error out"=w3325:errorcluster)  [unwired: 10 in]
                                n1788 = local write "data file error"(w3325) -> ()
                              }
                              frame #1 {
                                n1789 = Bundle("STATUS"=w3332, "OUT SERVER ADDRESS"=w3331, "FROM ACCOUNT"=w3330, "Mail Test File To:"=w3329, "Mail Test Fail"=w3328) -> (w3334:T32)  [unwired: 1 in]
                                n1790 = call "Save data file (pass-fail) v5.vi"("Input Cluster"=w3334, "panel id"=w3327) -> ("network file save error"=w3333:errorcluster)  [unwired: 8 in, 1 out]
                                n1791 = local write "data file error"(w3333) -> ()
                              }
                            }
                          }
                        }
                      }
                    }
                  }
                }
              }
              frame #8 {
                # "LAB05-1"
                n1792 = local read "run lab05-1"() -> (w3339:bool)
                n1793 = case shown="True" w3339 {
                  tunnel: w3338 -> [_ w3344]
                  tunnel: w3337 -> [_ w3343]
                  tunnel: w3336 -> [_ w3342]
                  tunnel: w3335 -> [_ w3341]
                  frame False {
                  }
                  frame True {
                    n1794 = local read "DISP LAB05-1"() -> (w3340:T4)
                    n1795 = Unbundle(w3340) -> ("CYCLE"=w3348:dbl, "STATUS"=w3345:string)  [unwired: 1 out]
                    n1796 = global write "Global display 2.vi" "DISP LAB05-1"(w3340) -> ()
                    n1797 = Not Equal?(x=w3345, y="RUN") -> (x != y?=w3347:bool)
                    n1798 = local read "TDMS LAB05-1"() -> (w3351:refnum<k34>)
                    n1799 = Greater?(x=w3348, y=2.0) -> (0:w3349:bool)
                    n1800 = And(x=w3349, y=w3347) -> (x .and. y?=w3346:bool)
                    n1801 = case shown="True" w3346 {
                      tunnel: w3340 -> [_ w3359]
                      tunnel: w3351 -> [_ w3358]
                      tunnel: w3345 -> [_ w3357]
                      tunnel: w3344 -> [_ w3356]
                      tunnel: w3343 -> [_ w3355]
                      tunnel: w3342 -> [_ w3354]
                      tunnel: w3341 -> [_ w3353]
                      frame False {
                      }
                      frame True {
                        n1802 = stacked-sequence {
                          tunnel: w3359 -> [w3362 _ _]
                          tunnel: w3358 -> [_ w3364 _]
                          tunnel: w3357 -> [_ _ w3370]
